vi "IMU_read_FPGA_streaming_data.vi"(0 "停止":bool, 2 "Number of bytes":u16=10, 3 "波特率":T1=enum."460.8 kbps") -> (1 "数据":u8 format="%x")   [LabVIEW 2016]
uses:
  <vilib>/LabVIEW Targets/FPGA/cRIO/shared/nicrio_ModuleControls/nicrio_cRIO-9871_BaudRateEnum.ctl
  <vilib>/LabVIEW Targets/FPGA/cRIO/shared/nicrio_ModuleControls/nicrio_cRIO-9871_DataBitsEnum.ctl
  <vilib>/LabVIEW Targets/FPGA/cRIO/shared/nicrio_ModuleControls/nicrio_cRIO-9871_ParityEnum.ctl
  <vilib>/LabVIEW Targets/FPGA/cRIO/shared/nicrio_ModuleControls/nicrio_cRIO-9871_StopBitsEnum.ctl
  <vilib>/LabVIEW Targets/FPGA/cRIO/shared/nicrio_ModuleControls/nicrio_cRIO-9871_XcvrModeEnum.ctl
  <vilib>/rvi/Emulation/niFpgaGetClockAttributes.vi
  <vilib>/rvi/Emulation/niFpgaSctlEmulationGetInTimedLoop.vi
  <vilib>/rvi/Emulation/niFpgaEmulationReportErrorSimple.vi
  <vilib>/rvi/eio/common/nirviEmuTemplatePropertySet_noerrors.vi
  <vilib>/rvi/eio/common/nirviEmuTemplateMethod_errors.vi
  <vilib>/rvi/interface/RandomDataEmulation/niFpgaRandomDataHandleErrors.vi
  <vilib>/rvi/Emulation/niFpgaCriticalErrorInLSC.vi
  <vilib>/eio/EIOPropertyNode/EIOPropertyNode.xnode
  <vilib>/eio/EIOMethodNode/EIOMethodNode.xnode
  <vilib>/rvi/DataTransferAndStorage/Container/XNode/niFpgaContainer.xnode
  <vilib>/rvi/interface/RandomDataEmulation/nirviRandomDataFpgaReadWriteTemplate.vi
  <vilib>/rvi/eio/common/nirviEmuTemplatePropertyGet_errors.vi
  <vilib>/rvi/eio/common/nirviEmuTemplatePropertyGet_noerrors.vi
  <vilib>/rvi/eio/common/nirviEmuTemplatePropertySet_errors.vi
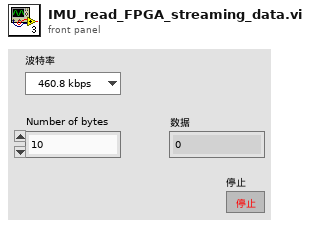
[diagram p1: front panel]
types:
  T1 = typedef "nicrio_cRIO-9871_BaudRateEnum.ctl" = enum16{"75 bps", "110 bps", "134 bps", "150 bps", "300 bps", "600 bps", "1200 bps", "1800 bps", "2400 bps", "4800 bps", "7200 bps", "9600 bps", "14.4 kbps", "19.2 kbps", "28.8 kbps", "38.4 kbps", "57.6 kbps", "115.2 kbps", "230.4 kbps", "460.8 kbps", "921.6 kbps"}
  T2 = typedef "nicrio_cRIO-9871_XcvrModeEnum.ctl" = enum8{"4 Wire", "2 Wire DTR Controlled with Echo", "2 Wire DTR Controlled", "2 Wire Auto"}
  T3 = typedef "nicrio_cRIO-9871_StopBitsEnum.ctl" = enum8{"1", "1.5", "2"}
  T4 = typedef "nicrio_cRIO-9871_ParityEnum.ctl" = enum8{"None", "Odd", "Even", "Mark", "Space"}
  T5 = typedef "nicrio_cRIO-9871_DataBitsEnum.ctl" = enum8{"5", "6", "7", "8"}
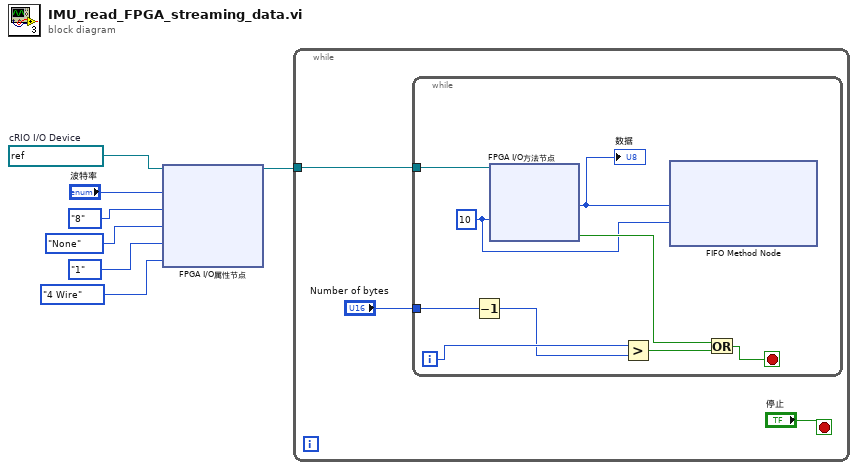
[diagram p0: block diagram]
diagram:
  w7 = refnum<k21> "模块3\\Port1"  # cRIO I/O Device
  n1 = xnode "FPGA I/O属性节点"("FPGA I/O In"=w7, "波特率"="波特率", "数据位"=nicrio_cRIO-9871_DataBitsEnum."8", "校验"=nicrio_cRIO-9871_ParityEnum."None", "停止位"=nicrio_cRIO-9871_StopBitsEnum."1", "收发器模式"=nicrio_cRIO-9871_XcvrModeEnum."4 Wire") -> ("FPGA I/O Out"=w1:refnum<k21>)
  n2 = while {
    tunnel: w1 -> [w9]
    stop <- "停止" stop-if-true
    n3 = while {
      tunnel: w9 -> [w19]
      tunnel: "Number of bytes" -> [w14]
      i -> [w18]
      stop <- w15 stop-if-true
      w11 = 10 ("超时(ms)")
      n4 = Decrement(x=w14) -> (x-1=w13:u16)
      n5 = xnode "FPGA I/O方法节点"("FPGA I/O In"=w19, "超时(ms)"=w11) -> ("数据"=w12:u8, "超时"=w17:bool)  [unwired: 1 out]
      "数据" <- w12
      n6 = Greater?(x=w18, y=w13) -> (0:w16:bool)
      n7 = xnode ("FIFO Method Node")("元素"=w12, "超时"=w11) -> ()  [unwired: 1 in, 2 out]
      n8 = Or(x=w17, y=w16) -> (x .or. y?=w15:bool)
    }
  }
